vi "AddTestCase.vi"(8 "error in (no error)":errorcluster, 9 "Name":string, 10 "Parent Tag (\"\")":string, 11 "ResultTree in":refnum<class "ResultTree.lvclass">) -> (0 "error out":errorcluster, 2 "Tag":string, 3 "ResultTree out":refnum<class "ResultTree.lvclass">)   [LabVIEW 2017, in "ResultTree.lvclass"]
doc: "Adds a test case. Returns the tag name."
uses:
  ResultTree.lvclass
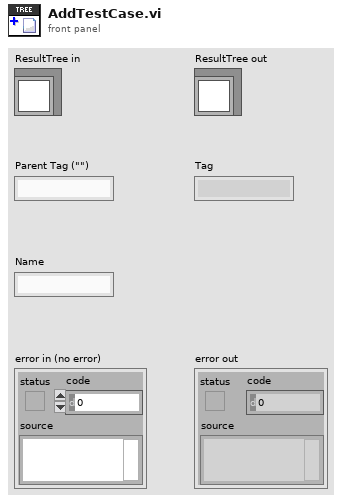
[diagram p1: front panel]
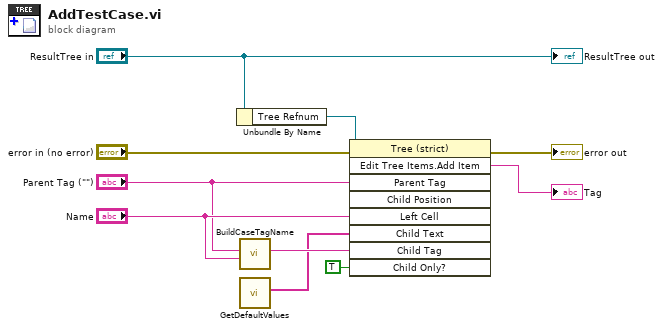
[diagram p0: block diagram]
diagram:
  n1 = Unbundle By Name("ResultTree in") -> ("Tree Refnum"=w7:refnum<vi>)
  n2 = call "BuildCaseTagName.vi"("Case Name"="Name", "Parent Tag"="Parent Tag (\"\")") -> ("Tag Name"=w6:string)  [unwired: 9 in]
  n3 = call "GetDefaultValues.vi"() -> ("Default Values"=w1:string[])  [unwired: 11 in]
  n4 = invoke class="Tree (strict)" method="Edit Tree Items.Add Item"(reference=w7, error in="error in (no error)", "Parent Tag"="Parent Tag (\"\")", "Left Cell"="Name", "Child Text"=w1, "Child Tag"=w6, "Child Only?"=TRUE) -> (error out=→"error out":errorcluster, "Edit Tree Items:Add Item"=→"Tag":string)  [unwired: 2 in, 7 out]
  "ResultTree out" <- "ResultTree in"
